vi "VCS Get Object_UINT64.vi"(0 "axis in":cluster{"keyHandle":u32, "nodeId":u16}={"keyHandle"=0, "nodeId"=1}, 5 "object in":T1 {"object subIndex" format="%x"; "object index" format="%x"}, 11 "error in (no error)":errorcluster) -> (4 "axis out":cluster{"keyHandle":u32, "nodeId":u16}={"keyHandle"=0, "nodeId"=1}, 6 "object out":T1 {"object subIndex" format="%x"; "object index" format="%x"}, 15 "error out":errorcluster)   [LabVIEW 2017, in "maxonEPOS.lvlib"]
doc: "<B>VCS GetObject</B> reads an UINT32 object value at the given index and sub index from object dictionary."
uses:
  Examples/maxonEPOS.lvlib
  SSI_Tool/InstrumentsInterfaces/Motordriver/maxon EPOS/Resources/EposCmd.dll
  SSI_Tool/InstrumentsInterfaces/Motordriver/maxon EPOS/Resources/EposCmd64.dll
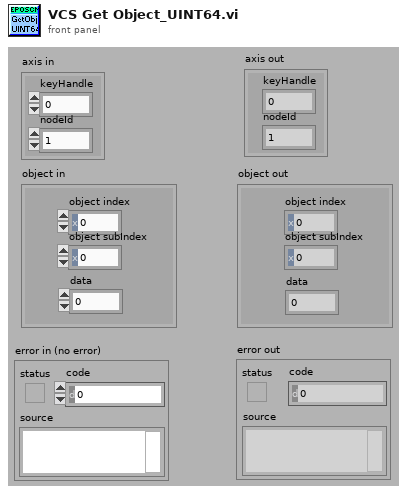
[diagram p1: front panel]
types:
  T1 = cluster{"object index":u16, "object subIndex":u8, "data":u32}
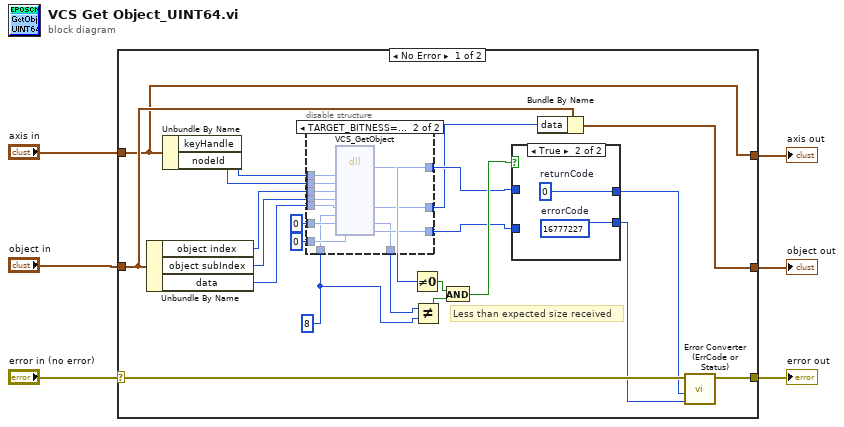
[diagram p0: block diagram]
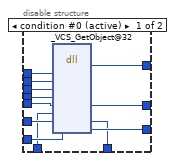
[diagram p2: hidden frame]
diagram:
  n1 = case shown="No Error" "error in (no error)" {
    selector: "error in (no error)" -> [w9 w59]
    tunnel: [w10 w59] -> w5
    tunnel: "axis in" -> [w16 w57]
    tunnel: "object in" -> [w17 w58]
    tunnel: [w19 w58] -> w3
    tunnel: [w16 w57] -> w1
    frame No Error {
      w12 = u32 8
      # "Less than expected size received"
      n2 = Unbundle By Name(w17) -> ("object index"=w18:u16, "object subIndex"=w26:u8, "data"=w13:u32)
      n3 = Unbundle By Name(w16) -> ("keyHandle"=w28:u32, "nodeId"=w27:u16)
      n4 = disable-structure shown="TARGET_BITNESS==64" {
        disable-tunnel: w28 -> [w40 w52]
        disable-tunnel: w27 -> [w39 w51]
        disable-tunnel: w26 -> [w38 w50]
        disable-tunnel: [w37 w49] -> w22
        disable-tunnel: [w36 w48] -> w21
        disable-tunnel: [w35 w47] -> w20
        disable-tunnel: w18 -> [w34 w46]
        disable-tunnel: u32 0 ("pNbOfBytesRead") -> [w33 w45]
        disable-tunnel: u32 0 ("pErrorCode") -> [w32 w44]
        disable-tunnel: w13 -> [w31 w43]
        disable-tunnel: w12 -> [w30 w42]
        disable-tunnel: [w29 w41] -> w11
        frame condition #0 (active) {
          n5 = dll-call lib="C:/workspace/project/scancon/sw/SSI_Tool/InstrumentsInterfaces/Motordriver/maxon EPOS/Resources/EposCmd.*" fn="_VCS_GetObject@32"("KeyHandle"=w40, "NodeId"=w39, "ObjectIndex"=w34, "ObjectSubIndex"=w38, "pData"=w31, "NbOfBytesToRead"=w30, "pNbOfBytesRead"=w33, "pErrorCode"=w32) -> (w35:i32, "pData"=w29:u32, "pNbOfBytesRead"=w36:u32, "pErrorCode"=w37:u32)  [unwired: 8 in, 2 out]
        }
        frame condition #1 {
          n6 = dll-call lib="C:/setup/Resources/EposCmd64.*" fn="VCS_GetObject" ("EposCmd.dll:_VCS_GetObject@32")("KeyHandle"=w52, "NodeId"=w51, "ObjectIndex"=w46, "ObjectSubIndex"=w50, "pData"=w43, "NbOfBytesToRead"=w42, "pNbOfBytesRead"=w45, "pErrorCode"=w44) -> ("Rückgabetyp"=w47:i32, "pData"=w41:u32, "pNbOfBytesRead"=w48:u32, "pErrorCode"=w49:u32)  [unwired: 8 in, 2 out]
        }
      }
      n7 = Not Equal To 0?(x=w20) -> (x != 0?=w24:bool)
      n8 = Not Equal?(x=w21, y=w12) -> (x != y?=w25:bool)
      n9 = And(x=w24, y=w25) -> (x .and. y?=w23:bool)
      n10 = case shown="True" w23 {
        tunnel: [w54 w56] -> w7
        tunnel: [w53 w55] -> w8
        tunnel: w20 -> [w54 _]
        tunnel: w22 -> [w53 _]
        frame False {
        }
        frame True {
          w55 = u32 16777227  # errorCode
          w56 = 0  # returnCode
        }
      }
      n11 = Bundle By Name(cluster=w17, "data"=w11) -> (w19:T1)
      n12 = call "Error Converter (ErrCode or Status).vi"("error code"=w8, "return type"=w7, "error in (no error)"=w9) -> ("error out"=w10:errorcluster)  [unwired: 7 in]
    }
    frame Error {
    }
  }
  "error out" <- w5
  "axis out" <- w1
  "object out" <- w3
